vi "WRP Init Acquisition.vi"(8 "error in (no error)":errorcluster, 10 "block_RegionReady":u8, 11 "block_PointReady":u8) -> (0 "error out":errorcluster, 3 "function return":i32)   [LabVIEW 2018, in "SesWrapper.lvlib"]
doc: "int STDCALL WRP_InitAcquisition(const _bool block_PointReady, const _bool block_RegionReady);"
uses:
  SesWrapper.lvlib
  build/Debug/SESWrapper.dll
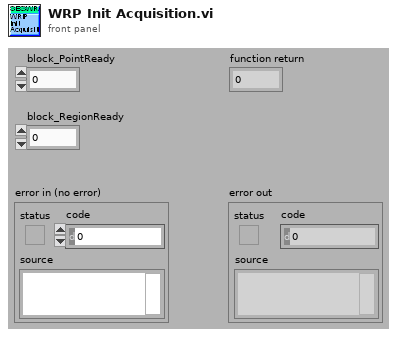
[diagram p1: front panel]
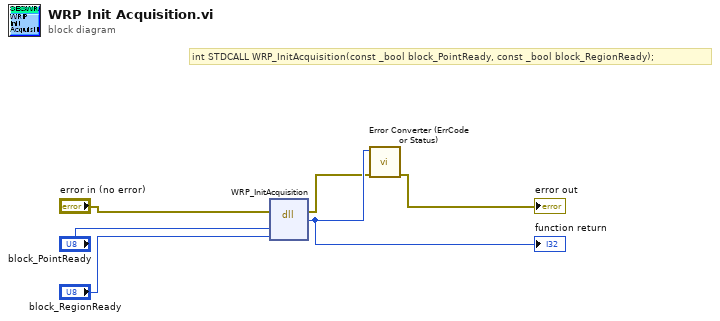
[diagram p0: block diagram]
diagram:
  # "int STDCALL WRP_InitAcquisition(const _bool block_PointReady, const _bool block_RegionReady);"
  n1 = dll-call lib="C:/Development/svn/seswrapper-lib/build/Debug/SESWrapper.*" fn="WRP_InitAcquisition"(error in="error in (no error)", "block_PointReady"="block_PointReady", "block_RegionReady"="block_RegionReady") -> (error out=w2:errorcluster, w6:i32)  [unwired: 4 in, 1 out]
  "function return" <- w6
  n2 = call "Error Converter (ErrCode or Status).vi"("error in (no error)"=w2, "error code"=w6) -> ("error out"=→"error out":errorcluster)  [unwired: 9 in]
